vi "set_date_and_create_initial_memory_image.vi"(0 "input cluster":T3) -> (1 "Acquired Buffer Number":u32, 2 "sub_directory":string)   [LabVIEW 2010]
uses:
  <vilib>/userDefined/High Color/IMAQdx.ctl
  <vilib>/vision/Image Controls.llb/IMAQ Image.ctl
  MWT_1.3.0_r1035/MultiWorm Tracker v1.3.0/data/MWT.dll
panel:
  out "return type 4":i32
  out "return type 3":i32
  out "return type 2":i32
  out "return type":i32
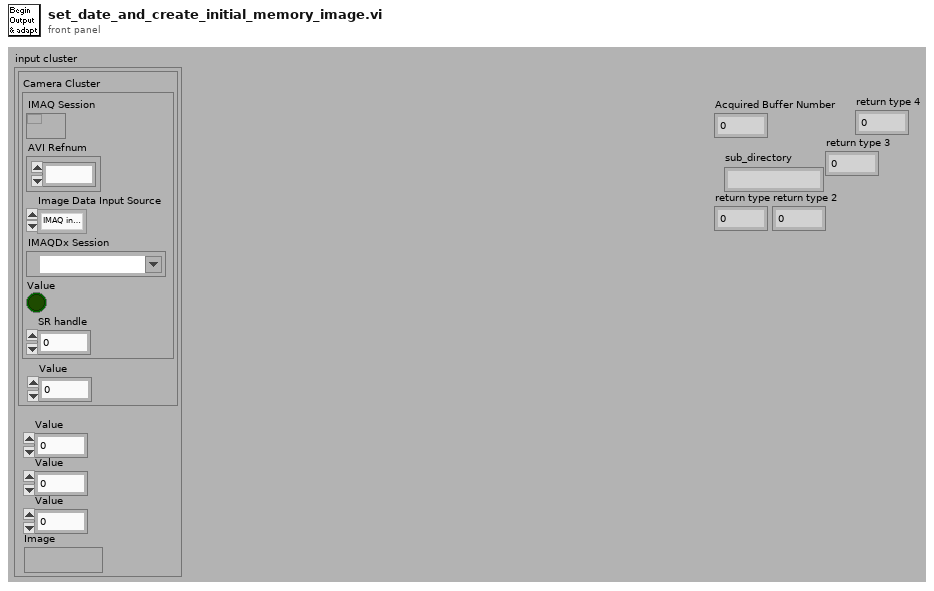
[diagram p1: front panel]
types:
  T1 = typedef "IMAQdx.ctl" = refnum<k21>
  T2 = typedef "IMAQ Image.ctl" = refnum<image>
  T3 = cluster{cluster{"Camera Cluster":cluster{"IMAQ Session":refnum<k11>, "AVI Refnum":refnum<k1>, "Image Data Input Source":enum32{"IMAQ interface", "IMAQdx interface", "AVI file", "MMF File"}, "IMAQDx Session":T1, "Value":bool, "SR handle":u32}, "Value":i32}, "Value":i32, "Value":i32, "Value":u16, "Image":T2}
  T4 = cluster{"Camera Cluster":cluster{"IMAQ Session":refnum<k11>, "AVI Refnum":refnum<k1>, "Image Data Input Source":enum32{"IMAQ interface", "IMAQdx interface", "AVI file", "MMF File"}, "IMAQDx Session":T1, "Value":bool, "SR handle":u32}, "Value":i32}
  T5 = typedef "LVDateTimeRec.ctl" = cluster{"fractional second":dbl, "second":i32, "minute":i32, "hour":i32, "day of month":i32, "month":i32, "year":i32, "day of week":i32, "day of year":i32, "DST":i32}
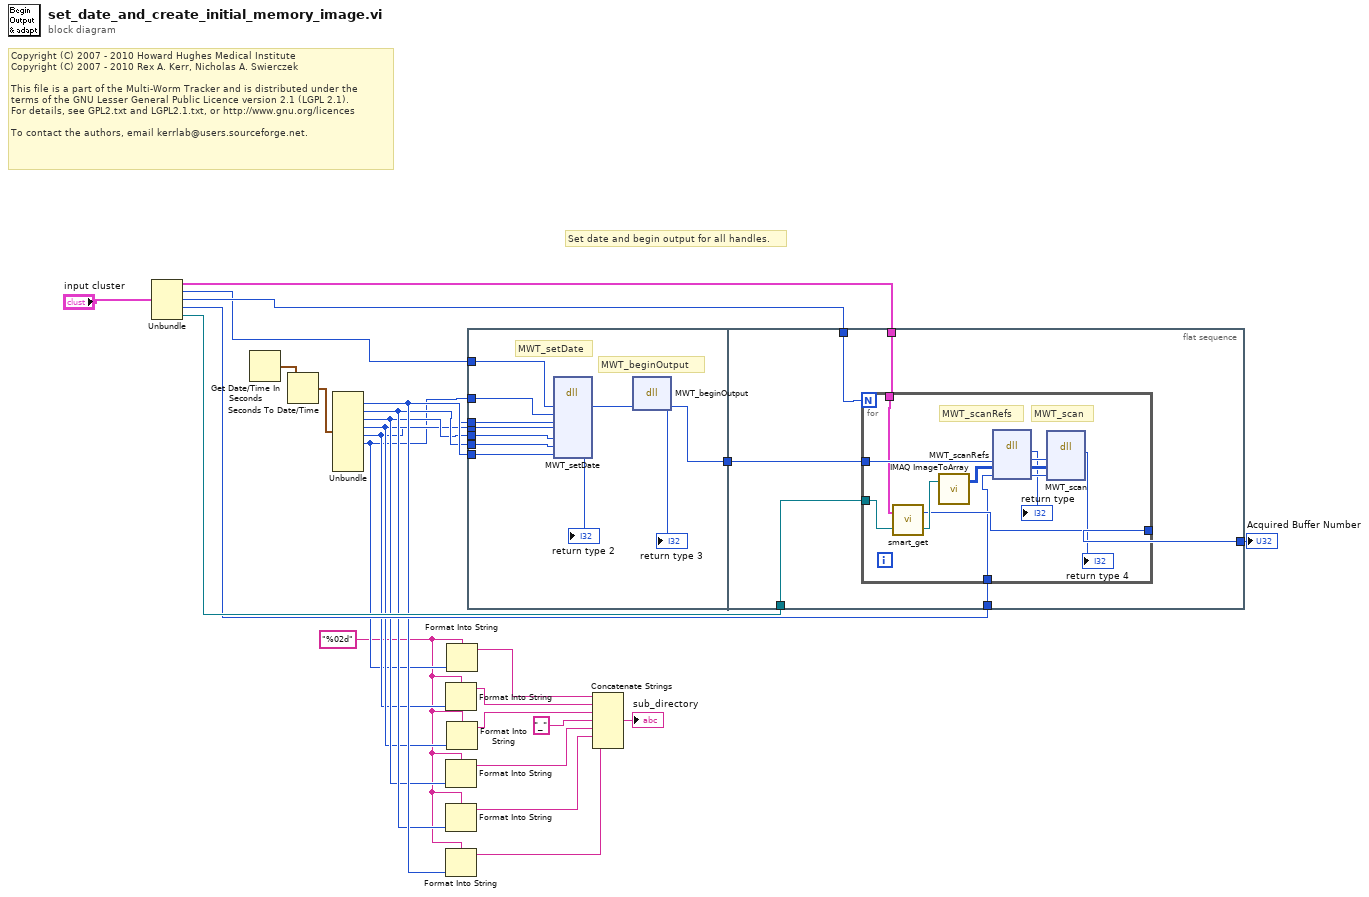
[diagram p0: block diagram]
diagram:
  w2 = "%02d" ("format string")
  # "Copyright (C) 2007 - 2010 Howard Hughes Medical Institute\nCopyright (C) 2007 - 2010 Rex A. Kerr, Nicholas A. Swierczek\n \nThis file is a part of the Multi-Worm Tracker and is distributed under the\nterms of the GNU Lesser General Public Licence version 2.1 (LGPL 2.1).\nFor details, see GPL2.txt and LGPL2.1.txt, or http://www.gnu.org/licences\n \nTo contact the authors, email kerrlab@users.sourceforge.net."
  # "Set date and begin output for all handles."
  n1 = Unbundle("input cluster") -> (w20:T4, "Value"=w17:i32, "Value"=w18:i32, "Value"=w19:u16, "Image"=w21:T2)
  n2 = Get Date/Time In Seconds() -> (seconds since 1Jan1904=w25:timestamp)
  n3 = Seconds To Date/Time(time stamp (now)=w25) -> (date time rec=w24:T5)  [unwired: 1 in]
  n4 = Unbundle(w24) -> ("second"=w16:i32, "minute"=w15:i32, "hour"=w14:i32, "day of month"=w13:i32, "month"=w12:i32, "year"=w11:i32)  [unwired: 4 out]
  n5 = Format Into String(format string=w2, w12) -> (resulting string=w9:string)  [unwired: 2 in, 1 out]
  n6 = Format Into String(format string=w2, w14) -> (resulting string=w6:string)  [unwired: 2 in, 1 out]
  n7 = Format Into String(format string=w2, w15) -> (resulting string=w5:string)  [unwired: 2 in, 1 out]
  n8 = Format Into String(format string=w2, w16) -> (resulting string=w4:string)  [unwired: 2 in, 1 out]
  n9 = Format Into String(format string=w2, w11) -> (resulting string=w10:string)  [unwired: 2 in, 1 out]
  n10 = Format Into String(format string=w2, w13) -> (resulting string=w8:string)  [unwired: 2 in, 1 out]
  n11 = flat-sequence {
    tunnel: w17 -> [w36]
    tunnel: w16 -> [w35]
    tunnel: w15 -> [w34]
    tunnel: w14 -> [w33]
    tunnel: w13 -> [w32]
    tunnel: w12 -> [w31]
    tunnel: w11 -> [w30]
    tunnel: [w28] -> w23
    tunnel: w21 -> [w37]
    tunnel: w23 -> [w42]
    tunnel: w18 -> [w41]
    tunnel: w19 -> [w40]
    tunnel: [w39] -> w22
    tunnel: w20 -> [w38]
    frame #0 {
      # "MWT_beginOutput"
      # "MWT_setDate"
      n12 = dll-call lib="C:/Users/Marc/multi worm tracker/MWT_1.3.0_r1035/MultiWorm Tracker v1.3.0/data/MWT.dll" fn="MWT_setDate"("handle"=w36, "year"=w30, "month"=w31, "day"=w32, "hour"=w33, "minute"=w34, "second"=w35) -> ("return type"=→"return type 2":i32, "handle"=w29:i32)  [unwired: 9 in, 2 out]
      n13 = dll-call lib="C:/Users/Marc/multi worm tracker/MWT_1.3.0_r1035/MultiWorm Tracker v1.3.0/data/MWT.dll" fn="MWT_beginOutput"("handle"=w29) -> ("return type"=→"return type 3":i32, "handle"=w28:i32)  [unwired: 3 in, 2 out]
    }
    frame #1 {
      n14 = for {
        N: w41 -> [_]
        tunnel: w37 -> [w52]
        tunnel: w42 -> [w46]
        tunnel: w40 -> [w48]
        tunnel: [w53] -> w39
        tunnel: w38 -> [w43]
        # "MWT_scanRefs"
        # "MWT_scan"
        n15 = call "smart_get.vi"("Input Image"=w52, "Cluster"=w43) -> ("Image Out"=w54:T2, "Acquired Buffer Number"=w53:i32)
        n16 = call "IMAQ ImageToArray"("Image"=w54) -> ("Image Pixels (I16)"=w47:i16[][])  [unwired: 3 in, 4 out]
        n17 = dll-call lib="C:/Users/Marc/multi worm tracker/MWT_1.3.0_r1035/MultiWorm Tracker v1.3.0/data/MWT.dll" fn="MWT_scanRefs"("handle"=w46, "image"=w47, "binning"=w48) -> ("return type"=→"return type":i32, "handle"=w51:i32, "image"=w50:i16[][], "binning"=w49:i32)  [unwired: 3 in, 2 out]
        n18 = dll-call lib="C:/Users/Marc/multi worm tracker/MWT_1.3.0_r1035/MultiWorm Tracker v1.3.0/data/MWT.dll" fn="MWT_scan"("handle"=w51, "image"=w50, "binning"=w49) -> ("return type"=→"return type 4":i32)  [unwired: 6 in, 2 out]
      }
    }
  }
  n19 = Concatenate Strings(w10, w9, w8, "_", w6, w5, w4) -> (→"sub_directory":string)
  "Acquired Buffer Number" <- w22
